vi "Logging Values (SubVI).vi"(8 "error in (no error)":errorcluster, 10 "Array":dbl[](array[numeric]) format="%#.1f", 11 "Byte Stream File in":refnum<file>) -> (0 "error out":errorcluster, 3 "Byte Stream File out":refnum<file>)   [LabVIEW 2014]
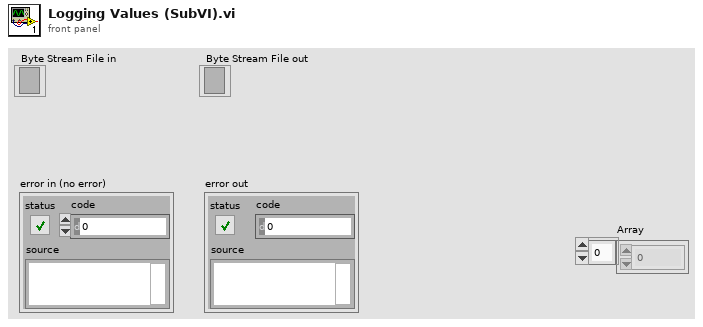
[diagram p1: front panel]
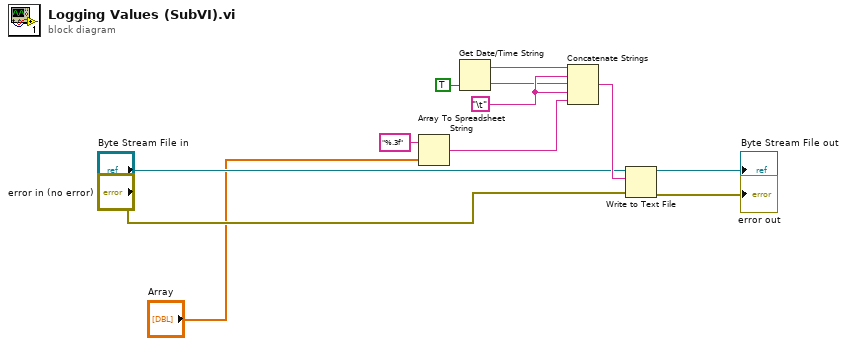
[diagram p0: block diagram]
diagram:
  w10 = "\t"
  n1 = Array To Spreadsheet String(array="Array", 3:"%.3f" ("format string")) -> (spreadsheet string=w11:string)  [unwired: 1 in]
  n2 = Get Date/Time String(want seconds? (F)=TRUE) -> (date string=w8:string, time string=w9:string)  [unwired: 2 in]
  n3 = Concatenate Strings(w8, w10, w9, w10, w11) -> (w12:string)
  n4 = Write to Text File(file (use dialog)="Byte Stream File in", text=w12, error in="error in (no error)") -> (refnum out=→"Byte Stream File out":refnum<file>, error out=→"error out":errorcluster)  [unwired: 1 in, 1 out]
